vi "debuggable read input.vi"(8 "error in":errorcluster, 10 "data table in in":T1, 11 "UDP Broadcaster Runtime in":refnum<class "TEC runtime.lvclass">) -> (0 "error out":errorcluster, 2 "data table out":T1, 3 "UDP Broadcaster Runtime out":refnum<class "TEC runtime.lvclass">)   [LabVIEW 2013, in "TEC runtime.lvclass"]
uses:
  TEC runtime.lvclass
  <vilib>/NI/Tag Bus/table/data table.ctl
  TEC runtime.lvclass/TEC runtime.ctl
  <vilib>/NI/Tag Bus/table/data table.lvlib
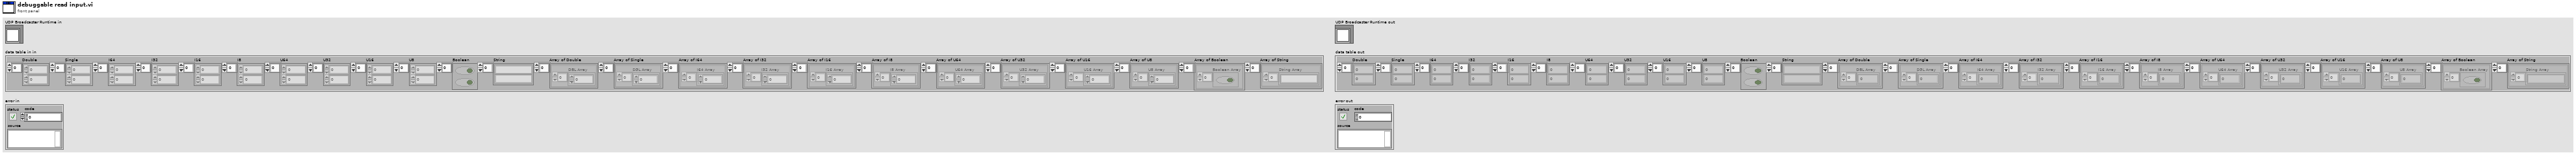
[diagram p1: front panel]
types:
  T1 = typedef "tag bus.lvlib/data table.lvlib/data table.ctl" = cluster{"Double":dbl[], "Single":sgl[], "I64":i64[], "I32":i32[], "I16":i16[], "I8":i8[], "U64":u64[], "U32":u32[], "U16":u16[], "U8":u8[], "Boolean":bool[], "String":string[], "Array of Double":cluster{"DBL Array":dbl[]}[], "Array of Single":cluster{"SGL Array":sgl[]}[], "Array of I64":cluster{"I64 Array":i64[]}[], "Array of I32":cluster{"I32 Array":i32[]}[], "Array of I16":cluster{"I16 Array":i16[]}[], "Array of I8":cluster{"I8 Array":i8[]}[], "Array of U64":cluster{"U64 Array":u64[]}[], "Array of U32":cluster{"U32 Array":u32[]}[], "Array of U16":cluster{"U16 Array":u16[]}[], "Array of U8":cluster{"U8 Array":u8[]}[], "Array of Boolean":cluster{"Boolean Array":bool[]}[], "Array of String":cluster{"String Array":string[]}[]}
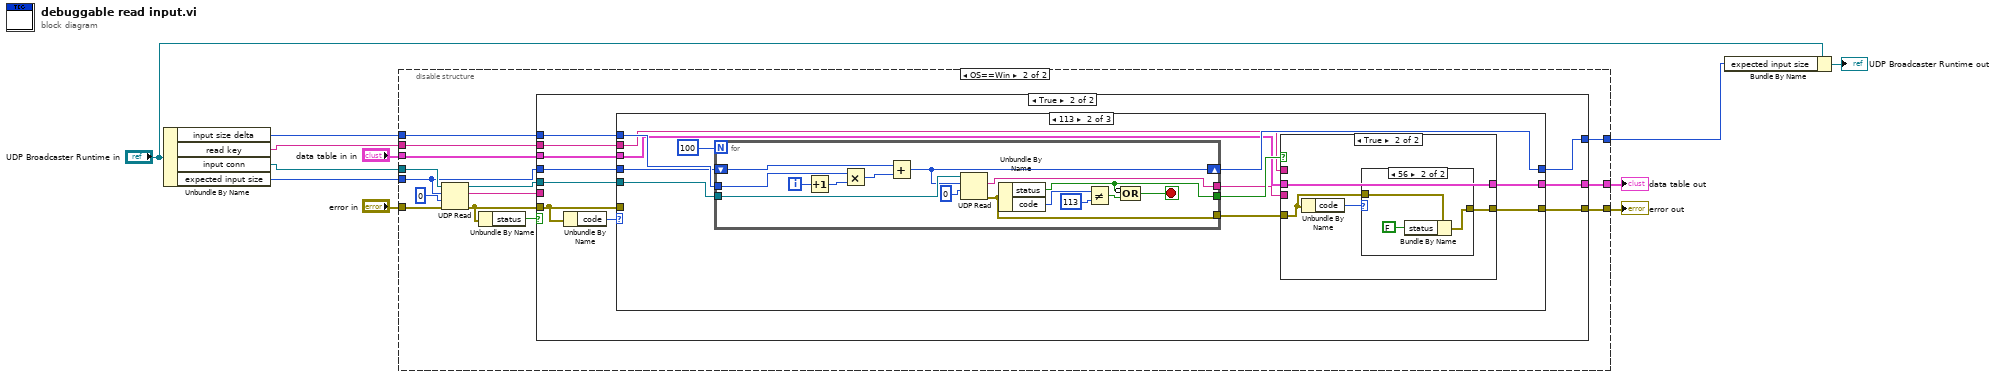
[diagram p0: block diagram]
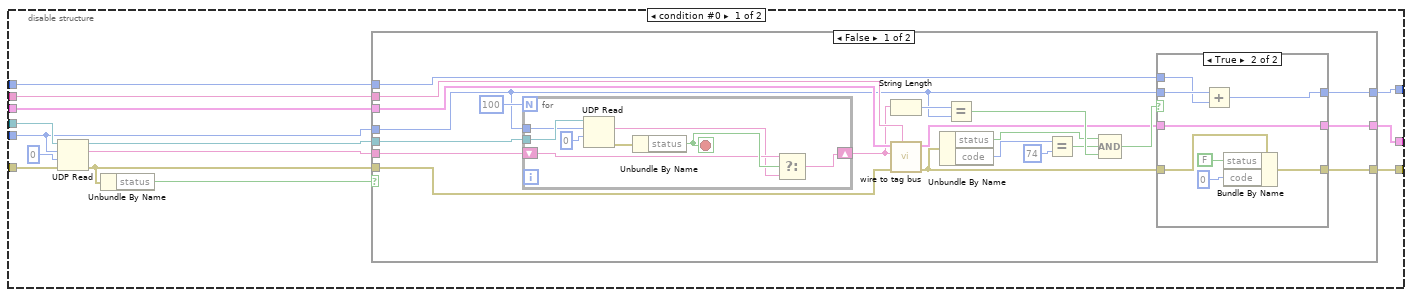
[diagram p2: hidden frame]
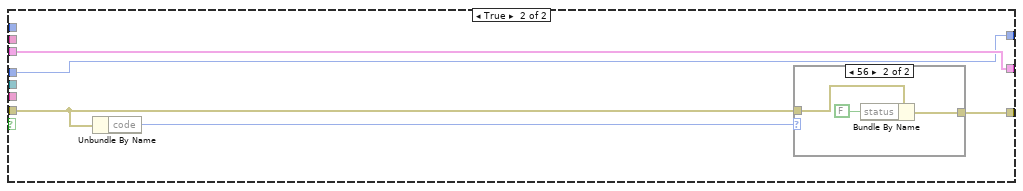
[diagram p4: hidden frame]
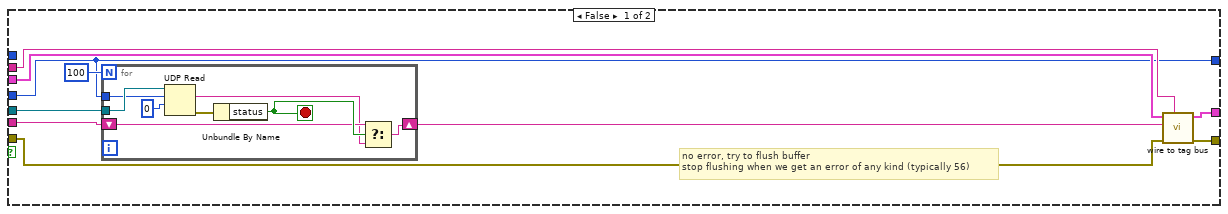
[diagram p6: hidden frame]
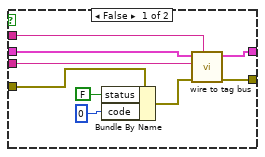
[diagram p8: hidden frame]
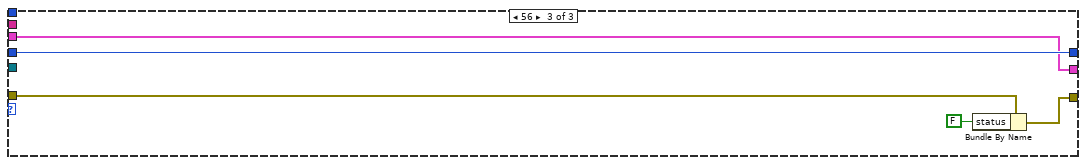
[diagram p10: hidden frame]
diagram:
  n1 = Unbundle By Name("UDP Broadcaster Runtime in") -> ("input size delta"=w8:i32, "read key"=w7:string, "input conn"=w1:refnum<k16>, "expected input size"=w6:i32)
  n2 = disable-structure shown="OS==Win" {
    disable-tunnel: w1 -> [w25 w87]
    disable-tunnel: "error in" -> [w23 w88]
    disable-tunnel: "data table in in" -> [w22 w78]
    disable-tunnel: [w21 w80] -> w4
    disable-tunnel: [w20 w79] -> w5
    disable-tunnel: w6 -> [w15 w76]
    disable-tunnel: w7 -> [w14 w82]
    disable-tunnel: w8 -> [w12 w75]
    disable-tunnel: [w13 w77] -> w10
    frame condition #0 {
      n3 = UDP Read(connection ID=w25, max size (548)=w15, timeout ms (25000)=0, 8:w23) -> (data out=w19:string, error out=w17:errorcluster, 3:w16:refnum<k16>)  [unwired: 2 out]
      n4 = Unbundle By Name(w17) -> ("status"=w18:bool)
      n5 = case shown="False" w18 {
        tunnel: w22 -> [w46 w67]
        tunnel: [w30 w68] -> w21
        tunnel: [w32 w67] -> w20
        tunnel: w19 -> [w44 _]
        tunnel: w17 -> [w42 w69]
        tunnel: w16 -> [w43 _]
        tunnel: w15 -> [w28 w66]
        tunnel: w14 -> [w41 _]
        tunnel: [w27 w66] -> w13
        tunnel: w12 -> [w26 _]
        frame False {
          n6 = for {
            N: 100 -> [_]
            shift-right: [w59] -> w40
            shift-left: w44 -> [w60]
            tunnel: w43 -> [w65]
            tunnel: w28 -> [w64]
            stop <- w61 stop-if-true
            n7 = UDP Read(connection ID=w65, max size (548)=w64, timeout ms (25000)=0) -> (data out=w58:string, error out=w62:errorcluster)  [unwired: 1 in, 3 out]
            n8 = Unbundle By Name(w62) -> ("status"=w61:bool)
            n9 = Select(t=w60, s=w61, f=w58) -> (s? t:f=w59:string)
          }
          n10 = String Length(string=w40) -> (length=w39:i32)
          n11 = call "wire to tag bus.vi"("unique key"=w41, "error in"=w42, "wire data"=w40, "data table in"=w46) -> ("error out"=w29:errorcluster, "data table out"=w31:T1)  [unwired: 6 in]
          n12 = Unbundle By Name(w29) -> ("status"=w34:bool, "code"=w38:i32)
          n13 = Equal?(x=w39, y=w28) -> (x = y?=w36:bool)
          n14 = Equal?(x=w38, y=74) -> (x = y?=w35:bool)
          n15 = Compound Arithmetic op=AND(w34, w35, w36) -> (w33:bool)
          n16 = case shown="True" w33 {
            tunnel: [w49 w57] -> w32
            tunnel: w31 -> [w49 w57]
            tunnel: [w48 w52] -> w30
            tunnel: w29 -> [w48 w53]
            tunnel: [w47 w54] -> w27
            tunnel: w28 -> [w47 w56]
            tunnel: w26 -> [_ w55]
            frame False {
            }
            frame True {
              n17 = Add(x=w56, y=w55) -> (x+y=w54:i32)
              n18 = Bundle By Name(cluster=w53, "status"=FALSE, "code"=0) -> (w52:errorcluster)
            }
          }
        }
        frame True {
          n19 = Unbundle By Name(w69) -> ("code"=w70:i32)
          n20 = case shown="56" w70 {
            tunnel: w69 -> [w71 w74]
            tunnel: [w71 w72] -> w68
            frame Default {
            }
            frame 56 {
              n21 = Bundle By Name(cluster=w74, "status"=FALSE) -> (w72:errorcluster)
            }
          }
        }
      }
    }
    frame condition #1 (active) {
      n22 = UDP Read(connection ID=w87, max size (548)=w76, timeout ms (25000)=0, 8:w88) -> (data out=w83:string, error out=w81:errorcluster, 3:w84:refnum<k16>)  [unwired: 2 out]
      n23 = Unbundle By Name(w81) -> ("status"=w85:bool)
      n24 = case shown="True" w85 {
        tunnel: w84 -> [w97 w109]
        tunnel: w83 -> [w96 _]
        tunnel: w82 -> [w94 w107]
        tunnel: w81 -> [w93 w115]
        tunnel: [w92 w114] -> w80
        tunnel: [w91 w110] -> w79
        tunnel: w78 -> [w90 w111]
        tunnel: [w89 w112] -> w77
        tunnel: w76 -> [w89 w113]
        tunnel: w75 -> [_ w108]
        frame False {
          # "no error, try to flush buffer\nstop flushing when we get an error of any kind (typically 56)"
          n25 = for {
            N: 100 -> [_]
            shift-right: [w101] -> w95
            shift-left: w96 -> [w102]
            tunnel: w97 -> [w106]
            tunnel: w89 -> [w99]
            stop <- w103 stop-if-true
            n26 = UDP Read(connection ID=w106, max size (548)=w99, timeout ms (25000)=0) -> (data out=w100:string, error out=w104:errorcluster)  [unwired: 1 in, 3 out]
            n27 = Unbundle By Name(w104) -> ("status"=w103:bool)
            n28 = Select(t=w102, s=w103, f=w100) -> (s? t:f=w101:string)
          }
          n29 = call "wire to tag bus.vi"("unique key"=w94, "error in"=w93, "wire data"=w95, "data table in"=w90) -> ("error out"=w92:errorcluster, "data table out"=w91:T1)  [unwired: 6 in]
        }
        frame True {
          n30 = Unbundle By Name(w115) -> ("code"=w116:i32)
          n31 = case shown="113" w116 {
            tunnel: [w118 w125 w167] -> w114
            tunnel: w115 -> [w118 _ w166]
            tunnel: w113 -> [w119 w128 w165]
            tunnel: [w119 w127 w165] -> w112
            tunnel: w111 -> [w117 w124 w164]
            tunnel: [w117 w123 w164] -> w110
            tunnel: w109 -> [_ w130 _]
            tunnel: w108 -> [_ w129 _]
            tunnel: w107 -> [_ w122 _]
            frame Default {
            }
            frame 113 {
              n32 = for {
                N: 100 -> [_]
                tunnel: w130 -> [w163]
                tunnel: w129 -> [w159]
                shift-right: [w156] -> w127
                shift-left: w128 -> [w157]
                tunnel: [w155] -> w121
                tunnel: [w150] -> w126
                tunnel: [w149] -> w120
                i -> [w161]
                stop <- w151 stop-if-true
                n33 = Increment(x=w161) -> (x+1=w160:i32)
                n34 = Multiply(x=w159, y=w160) -> (x*y=w158:i32)
                n35 = Add(x=w157, y=w158) -> (x+y=w156:i32)
                n36 = UDP Read(connection ID=w163, max size (548)=w156, timeout ms (25000)=0) -> (data out=w155:string, error out=w149:errorcluster)  [unwired: 1 in, 3 out]
                n37 = Unbundle By Name(w149) -> ("status"=w150:bool, "code"=w154:i32)
                n38 = Not Equal?(x=w154, y=113) -> (x != y?=w152:bool)
                n39 = Compound Arithmetic op=OR(invert w150, w152) -> (w151:bool)
              }
              n40 = case shown="True" w126 {
                tunnel: [w137 w141] -> w125
                tunnel: w124 -> [w136 w144]
                tunnel: [w135 w144] -> w123
                tunnel: w122 -> [w134 _]
                tunnel: w121 -> [w133 _]
                tunnel: w120 -> [w132 w142]
                frame False {
                  n41 = Bundle By Name(cluster=w132, "status"=FALSE, "code"=0) -> (w138:errorcluster)
                  n42 = call "wire to tag bus.vi"("unique key"=w134, "error in"=w138, "wire data"=w133, "data table in"=w136) -> ("error out"=w137:errorcluster, "data table out"=w135:T1)  [unwired: 6 in]
                }
                frame True {
                  n43 = Unbundle By Name(w142) -> ("code"=w143:i32)
                  n44 = case shown="56" w143 {
                    tunnel: w142 -> [w145 w147]
                    tunnel: [w145 w146] -> w141
                    frame Default {
                    }
                    frame 56 {
                      n45 = Bundle By Name(cluster=w147, "status"=FALSE) -> (w146:errorcluster)
                    }
                  }
                }
              }
            }
            frame 56 {
              n46 = Bundle By Name(cluster=w166, "status"=FALSE) -> (w167:errorcluster)
            }
          }
        }
      }
    }
  }
  "data table out" <- w5
  "error out" <- w4
  n47 = Bundle By Name(cluster="UDP Broadcaster Runtime in", "expected input size"=w10) -> (→"UDP Broadcaster Runtime out":refnum<class "TEC runtime.lvclass">)
